vi "PC_Rebin_Counts.vi"(9 "Bin time (ms)":dbl=1.0 min=0.001 max=50.0, 11 "Waveform in":waveform(i32)={"t0"=timestamp(0 s since 1904-01-01), "dt"=1e-06, "Y"=[]}) -> (3 "Waveform out":waveform(i32))   [LabVIEW 2020]
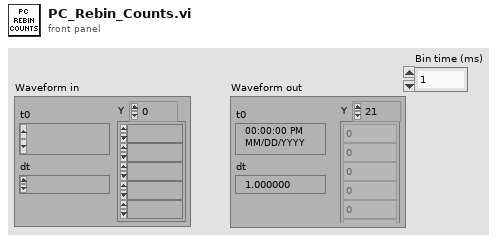
[diagram p1: front panel]
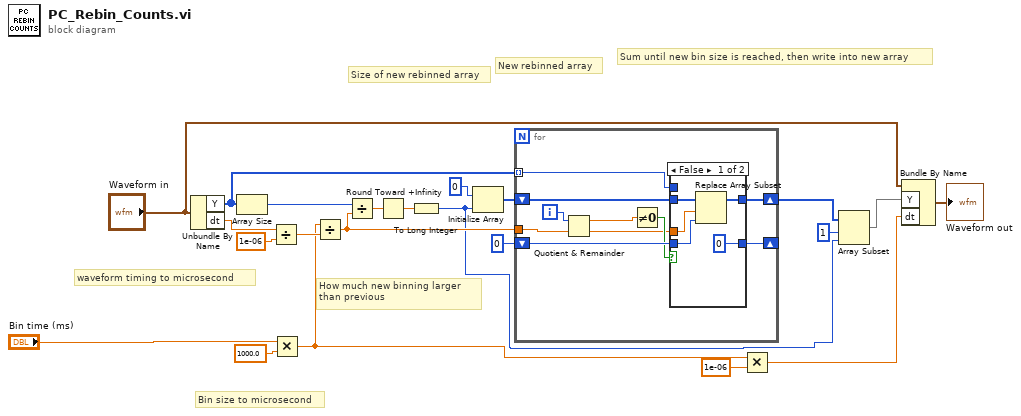
[diagram p0: block diagram]
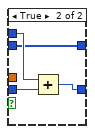
[diagram p2: hidden frame]
diagram:
  # "Sum until new bin size is reached, then write into new array"
  # "New rebinned array"
  # "Size of new rebinned array"
  # "How much new binning larger\nthan previous"
  # "waveform timing to microsecond"
  # "Bin size to microsecond"
  n1 = Unbundle By Name("Waveform in") -> ("Y"=w19:i32[], "dt"=w11:dbl)
  n2 = Array Size(array=w19) -> (size(s)=w17:i32)
  n3 = Divide(x=w11, y=1e-06) -> (x/y=w9:dbl)
  n4 = Multiply(x="Bin time (ms)", y=1000.0) -> (x*y=w7:dbl)
  n5 = Divide(x=w7, y=w9) -> (x/y=w8:dbl)
  n6 = Divide(x=w17, y=w8) -> (x/y=w16:dbl)
  n7 = Round Toward +Infinity(x=w16) -> (ceil(x): smallest int >= x=w15:dbl)
  n8 = To Long Integer(number=w15) -> (32bit integer=w1:i32)
  n9 = Initialize Array(0, w1) -> (w13:i32[])
  n10 = for {
    tunnel: w19 -> [w31] mode=indexing
    shift-right: [w30] -> _
    shift-left: 0 -> [w32]
    tunnel: w8 -> [w28]
    shift-right: [w23] -> w3
    shift-left: w13 -> [w25]
    i -> [w29]
    n11 = Quotient & Remainder(x=w29, y=w28) -> (x-y*floor(x/y)=w27:dbl, floor(x/y)=w24:dbl)
    n12 = Not Equal To 0?(x=w27) -> (x != 0?=w26:bool)
    n13 = case shown="False" w26 {
      tunnel: w32 -> [w34 w41]
      tunnel: w31 -> [_ w40]
      tunnel: [0 w39] -> w30
      tunnel: w25 -> [w36 w38]
      tunnel: w24 -> [w35 _]
      tunnel: [w33 w38] -> w23
      frame False {
        n14 = Replace Array Subset(array=w36, new element=w34, index=w35) -> (w33:i32[])
      }
      frame True {
        n15 = Add(x=w40, y=w41) -> (x+y=w39:i32)
      }
    }
  }
  n16 = Multiply(x=w7, y=1e-06) -> (x*y=w5:dbl)
  n17 = Array Subset(array=w3, index=1, length=w1) -> (w2:i32[])
  n18 = Bundle By Name(cluster="Waveform in", "Y"=w2, "dt"=w5) -> (→"Waveform out":waveform(i32))
